vi "wrap phase.vi"(11 "phase in (deg)":dbl) -> (3 "phase out (deg)":dbl)   [LabVIEW 2020]
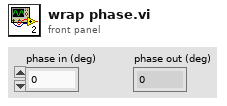
[diagram p1: front panel]
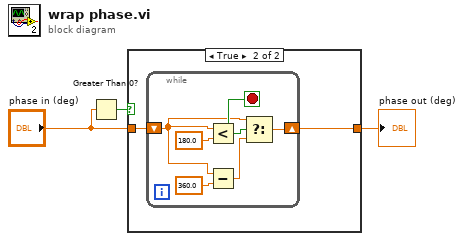
[diagram p0: block diagram]
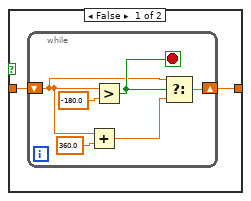
[diagram p2: hidden frame]
diagram:
  n1 = Greater Than 0?(x="phase in (deg)") -> (x > 0?=w3:bool)
  n2 = case shown="True" w3 {
    tunnel: [w4 w13] -> w2
    tunnel: "phase in (deg)" -> [w5 w12]
    frame False {
      n3 = while {
        shift-right: [w10] -> w4
        shift-left: w5 -> [w7]
        stop <- w9 stop-if-true
        n4 = Add(x=w7, y=360.0) -> (x+y=w8:dbl)
        n5 = Greater?(x=w7, y=-180.0) -> (0:w9:bool)
        n6 = Select(t=w7, s=w9, f=w8) -> (s? t:f=w10:dbl)
      }
    }
    frame True {
      n7 = while {
        shift-right: [w18] -> w13
        shift-left: w12 -> [w15]
        stop <- w17 stop-if-true
        n8 = Less?(x=w15, y=180.0) -> (x < y?=w17:bool)
        n9 = Subtract(x=w15, y=360.0) -> (x-y=w16:dbl)
        n10 = Select(t=w15, s=w17, f=w16) -> (s? t:f=w18:dbl)
      }
    }
  }
  "phase out (deg)" <- w2
